vi "CALC_CORR_STAT.vi"(0 "VISA IN":refnum<visa-resource-name>, 1 "Correction State ON/OFF":bool, 5 "error in":errorcluster, 7 "Channel":i32) -> (14 "VISA Out":refnum<visa-resource-name>, 19 "error out":errorcluster)   [LabVIEW 2018, in "PNA-X.lvlib"]
doc: "CALCulate<cnum>: CORRection:[STATe] <bool> \n1487\n\n(Read-Write) Turns error correction ON or OFF for the selected measurement on the specified \nchannel. \nTo turn error correction ON or OFF for a channel, use SENS:CORR:STATe. \nSee Critical Note \nParameters \n<cnum> Any existing channel number. If unspecified, value is set to 1 \n<bool> Correction state. Choose from: \n0 - Correction OFF \n1 - Correction ON \nExamples CALC:CORR ON \ncalculate:correction:state off \nQuery Syntax CALCulate<cnum>: CORRection: STATe? \nReturn Type Boolean \nDefault Not Applicable"
uses:
  PNA-X.lvlib
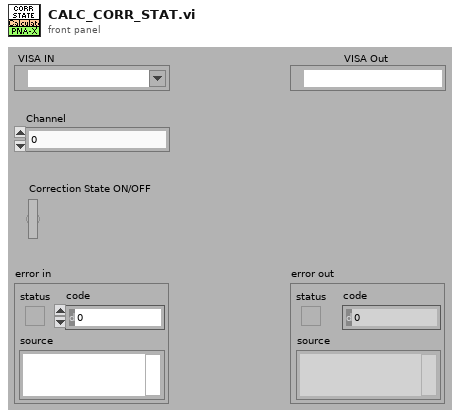
[diagram p1: front panel]
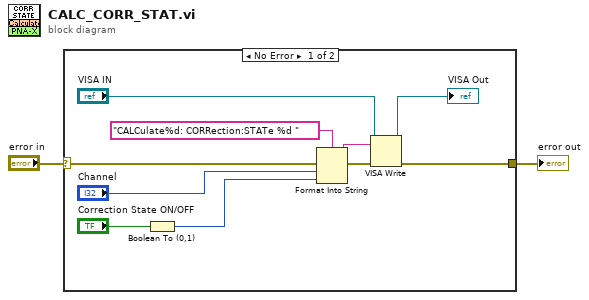
[diagram p0: block diagram]
diagram:
  n1 = case shown="No Error" "error in" {
    selector: "error in" -> [w12 w13]
    tunnel: [w7 w13] -> w1
    frame No Error {
      n2 = Boolean To (0,1)(Boolean="Correction State ON/OFF") -> (0, 1=w3:i16)
      n3 = Format Into String(format string="CALCulate%d: CORRection:STATe %d " ("Cmdline"), error in=w12, "Channel", w3) -> (resulting string=w10:string, error out=w11:errorcluster)  [unwired: 1 in]
      n4 = VISA Write(VISA resource name="VISA IN", write buffer=w10, error in (no error)=w11) -> (VISA resource name out=→"VISA Out":refnum<visa-resource-name>, error out=w7:errorcluster)  [unwired: 1 out]
    }
    frame Error {
    }
  }
  "error out" <- w1
